vi "Query Spectral Baseline Correction.vi"(8 "error in (no error)":errorcluster, 11 "VISA resource name":refnum<visa-resource-name>) -> (0 "error out":errorcluster, 2 "Spectral Baseline Correction":dbl, 3 "VISA resource name out":refnum<visa-resource-name>)   [LabVIEW 2019, in "Ocean Optics 2000 4000.lvlib"]
doc: "Returns the spectral baseline correction. This information is used to set the scale of each pixel's intensity value. \n\n<b>Note:</b>\nThis function is not supported by spectrometer model USB2000, HR4000, HR2000+,HR2000, MAYA, MAYA Pro and QE65000."
uses:
  Ocean Optics 2000 4000.lvlib
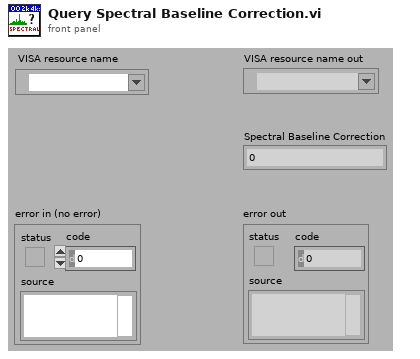
[diagram p1: front panel]
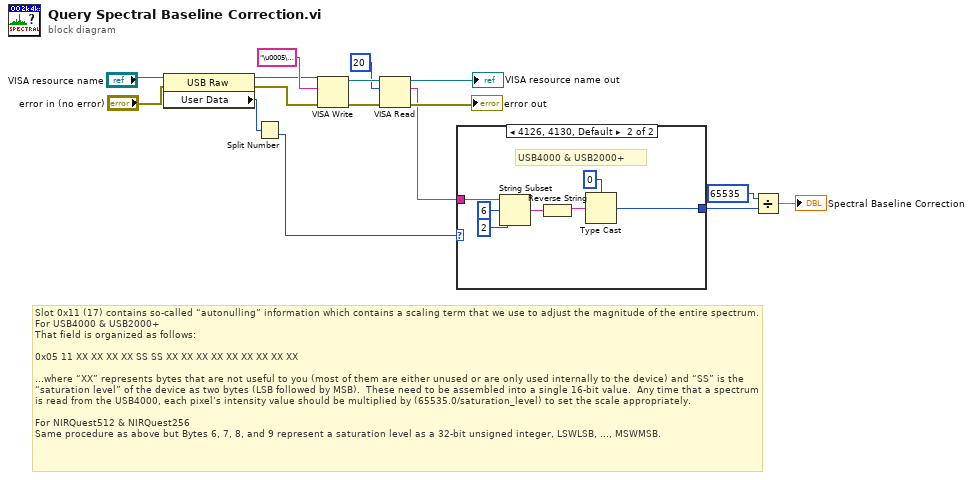
[diagram p0: block diagram]
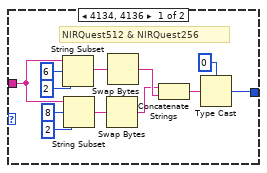
[diagram p2: hidden frame]
diagram:
  # "Slot 0x11 (17) contains so-called “autonulling” information which contains a scaling term that we use to adjust the magnitude of the entire spectrum.  \nFor USB4000 & USB2000+\nThat field is organized as follows: \n  \n0x05 11 XX XX XX XX SS SS XX XX XX XX XX XX XX XX XX \n  \n…where “XX” represents bytes that are not useful to you (most of them are either unused or are only used internally to the device) and “SS” is the “saturation level” of the device as two bytes (LSB followed by MSB).  These need to be assembled into a single 16-bit value.  Any time that a spectrum is read from the USB4000, each pixel’s intensity value should be multiplied by (65535.0/saturation_level) to set the scale appropriately. \n\nFor NIRQuest512 & NIRQuest256\nSame procedure as above but Bytes 6, 7, 8, and 9 represent a saturation level as a 32-bit unsigned integer, LSWLSB, …, MSWMSB."
  n1 = property class="USB Raw"(reference="VISA resource name", error in="error in (no error)") -> (reference out=w6:refnum<visa-resource-name>, error out=w5:errorcluster, "User Data"=w4:u32)
  n2 = Split Number(x=w4) -> (lo(x)=w3:u16)  [unwired: 1 out]
  n3 = VISA Write(VISA resource name=w6, write buffer="\u0005\u0011", error in (no error)=w5) -> (VISA resource name out=w14:refnum<visa-resource-name>, error out=w15:errorcluster)  [unwired: 1 out]
  n4 = VISA Read(VISA resource name=w14, byte count=u32 20, error in (no error)=w15) -> (VISA resource name out=→"VISA resource name out":refnum<visa-resource-name>, read buffer=w2:string, error out=→"error out":errorcluster)  [unwired: 1 out]
  n5 = case shown="4126, 4130, Default" w3 {
    tunnel: w2 -> [w24 w30]
    tunnel: [w19 w29] -> w1
    frame 4134, 4136 {
      # "NIRQuest512 & NIRQuest256"
      n6 = String Subset(string=w24, offset (0)=6, length (rest)=2 ("length (rest)")) -> (substring=w23:string)
      n7 = String Subset(string=w24, offset (0)=8, length (rest)=2 ("length (rest)")) -> (substring=w22:string)
      n8 = Swap Bytes(anything=w22) -> (byte swapped=w17:string)
      n9 = Swap Bytes(anything=w23) -> (byte swapped=w18:string)
      n10 = Concatenate Strings(w17, w18) -> (w20:string)
      n11 = Type Cast(type=u32 0, x=w20) -> (*(type *) &x=w19:u32)
    }
    frame 4126, 4130, Default {
      # "USB4000 & USB2000+"
      n12 = String Subset(string=w30, offset (0)=6, length (rest)=2 ("length (rest)")) -> (substring=w33:string)
      n13 = Reverse String(1:w33) -> (0:w34:string)
      n14 = Type Cast(type=u16 0, x=w34) -> (*(type *) &x=w29:u16)
    }
  }
  n15 = Divide(x=u32 65535, y=w1) -> (x/y=→"Spectral Baseline Correction":dbl)
